vi "Create DoubleMsg.vi"(8 "error in (no error)":errorcluster, 10 "Message Data":dbl, 11 "Message Name":string) -> (0 "error out":errorcluster, 3 "DoubleMsg Out":refnum<class "DoubleMsg.lvclass">)   [LabVIEW 2017, in "LapDog.Messaging.v3.NativeTypes.lvlib" / "DoubleMsg.lvclass"]
doc: "Returns a DoubleMsg object with the given name.\n\nThis method executes regardless of the error in state."
uses:
  DoubleMsg.lvclass
  C:/git/LapDog.Messaging/src/LapDog.Messaging/Message/Message.lvclass
  DoubleMsg.lvclass/DoubleMsg.ctl
  LapDog.Messaging/Message/Message.lvclass
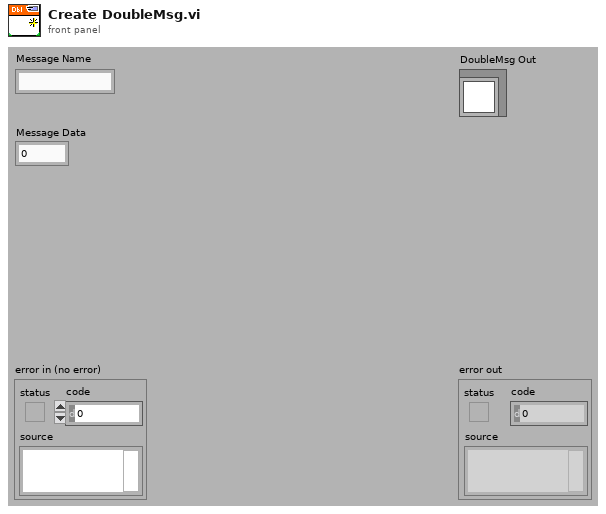
[diagram p1: front panel]
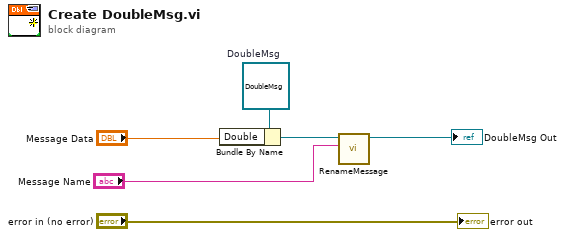
[diagram p0: block diagram]
diagram:
  w6 = refnum<class "DoubleMsg.lvclass"> refnum  # DoubleMsg
  n1 = Bundle By Name(cluster=w6, "Double"="Message Data") -> (w3:refnum<class "DoubleMsg.lvclass">)
  n2 = call "RenameMessage.vi"("Message Name"="Message Name", "Message in"=w3) -> ("Message out"=→"DoubleMsg Out":refnum<class "DoubleMsg.lvclass">)  [unwired: 8 in, 1 out]
  "error out" <- "error in (no error)"
